vi "User Comment Dialog.vi"(8 "error in":errorcluster, 10 "Timestamp":timestamp, 11 "M_Butt in":refnum<class "M_Butt.lvclass">) -> (0 "error out":errorcluster, 3 "M_Butt out":refnum<class "M_Butt.lvclass">)   [LabVIEW 2019, in "M_Butt.lvlib" / "M_Butt.lvclass"]
uses:
  Project/M_Butt.lvclass
  C:/Users/Public/Documents/Development/builds/Engine/Engine.lvlibp/Project/Engine.lvclass
  builds/Engine/Engine.lvlibp/Accessors/Read Report Queue.vi
  builds/Tools/QDMH.lvlibp/QDMH.lvclass
panel:
  in  "Cancel":bool
  in  "OK":bool caption="OK2"
  in  "Enter comment details and press 'Ok':":string
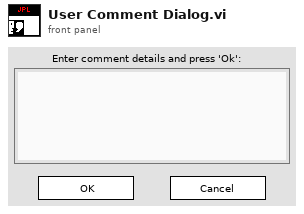
[diagram p1: front panel]
types:
  T1 = cluster{"Timestamp":timestamp, "Instrument":string, "Description":string, "Data":string}
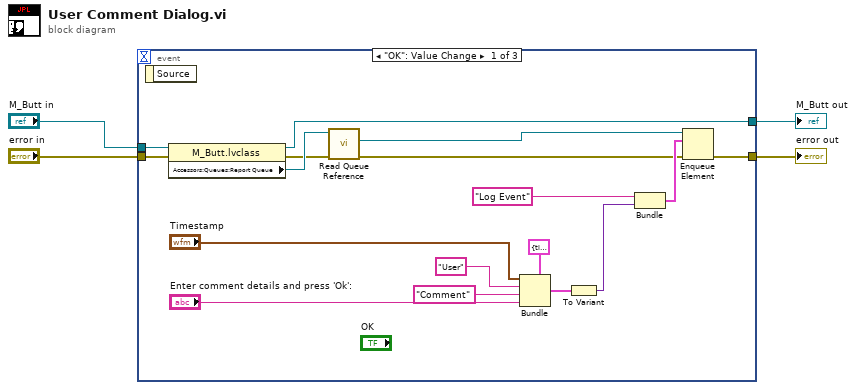
[diagram p0: block diagram]
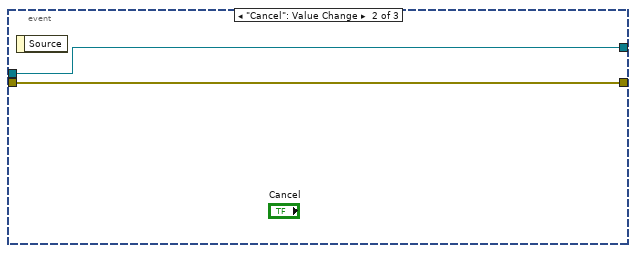
[diagram p2: hidden frame]
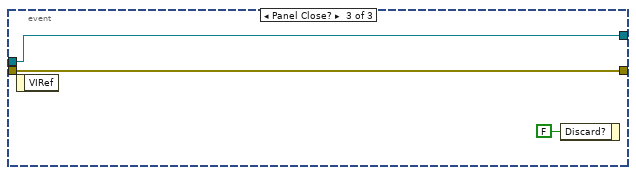
[diagram p3: hidden frame]
diagram:
  n1 = event shown="[0] \"OK\": Value Change" {
    selector: _ -> [_ _ _]
    dyn-events: _ -> [_ _ _]
    timeout: _ -> [_ _ _]
    tunnel: "M_Butt in" -> [w17 w23 w26]
    tunnel: [w16 w23 w26] -> w3
    tunnel: "error in" -> [w15 w22 w25]
    tunnel: [w9 w22 w25] -> w1
    event "OK": Value Change {
      n2 = event-data() -> ()  [unwired: 1 in, 1 out]
      n3 = property class="M_Butt.lvclass"(reference=w17, error in=w15) -> (reference out=w16:refnum<class "M_Butt.lvclass">, error out=w11:errorcluster, "Accessors:Queues:Report Queue"=w14:refnum<class "QDMH.lvclass">)
      n4 = call "Read Queue Reference.vi"("error in"=w11, "QDMH in"=w14) -> ("error out"=w10:errorcluster, "Queue Reference"=w13:refnum<queue>)  [unwired: 7 in, 1 out]
      n5 = Bundle(cluster=T1 {"Timestamp"=timestamp(0 s since 1904-01-01), "Instrument"="", "Description"="", "Data"=""} ("Event Data"), "Timestamp"="Timestamp", "Instrument"="User", "Description"="Comment", "Data"="Enter comment details and press 'Ok':") -> (w19:T1)
      n6 = To Variant(anything=w19) -> (Variant=w18:variant)
      n7 = Bundle("Log Event", "Variant"=w18) -> (w12:cluster{string, "Variant":variant})  [unwired: 1 in]
      n8 = Enqueue Element(queue=w13, element=w12, error in (no error)=w10) -> (error out=w9:errorcluster)  [unwired: 1 in, 2 out]
    }
    event "Cancel": Value Change {
      n9 = event-data() -> ()  [unwired: 1 in, 1 out]
    }
    event Panel Close? {
      n10 = event-data() -> ()  [unwired: 1 in, 1 out]
      n11 = event-data("Discard?"=FALSE) -> ()  [unwired: 1 in, 1 out]
    }
  }
  "error out" <- w1
  "M_Butt out" <- w3
